vi "RSZVB Diagram Area Delete.vi"(8 "error in (no error)":errorcluster {"code" format="%.0x"}, 10 "Window (1)":i32=1, 11 "VISA session":refnum<visa-resource-name>) -> (0 "error out":errorcluster {"code" format="%.0x"}, 3 "dup VISA session":refnum<visa-resource-name>)   [LabVIEW 2011]
doc: "This VI deletes a diagram area, identified by its area number <Wnd>.\n\nRemote-control command(s):\nDISPlay:WINDow<Wnd>:STATe OFF"
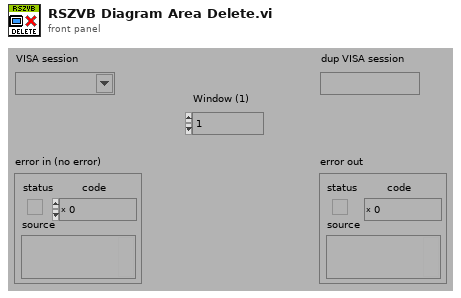
[diagram p1: front panel]
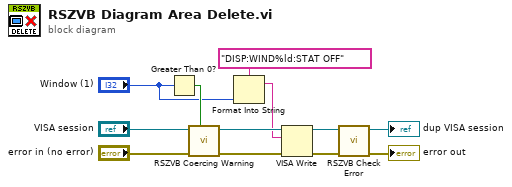
[diagram p0: block diagram]
diagram:
  n1 = Greater Than 0?(x="Window (1)") -> (x > 0?=w6:bool)
  n2 = call "RSZVB Coercing Warning.vi"("In Range?"=w6, "error in (no error)"="error in (no error)", "VISA session"="VISA session") -> ("error out"=w10:errorcluster, "dup VISA session"=w11:refnum<visa-resource-name>)  [unwired: 7 in]
  n3 = Format Into String(format string="DISP:WIND%ld:STAT OFF", "Window (1)") -> (resulting string=w7:string)  [unwired: 2 in, 1 out]
  n4 = VISA Write(VISA resource name=w11, write buffer=w7, error in (no error)=w10) -> (VISA resource name out=w8:refnum<visa-resource-name>, error out=w9:errorcluster)  [unwired: 1 out]
  n5 = call "RSZVB Check Error.vi"("error in (no error)"=w9, "VISA session"=w8) -> ("error out"=→"error out":errorcluster, "dup VISA session"=→"dup VISA session":refnum<visa-resource-name>)  [unwired: 8 in]
